vi "OP600ZP_ISO.vi"(8 "entrée d'erreur (pas d'erreur)":errorcluster, 9 "Oui":bool, 10 "reference en entrée":refnum<vi>) -> (0 "sortie d'erreur":errorcluster, 1 "ISOP":string, 2 "ISOM":string, 3 "Booléen":bool)   [LabVIEW 2020]
uses:
  VG/PackType.vi
  OP600ZP_VGConf.vi
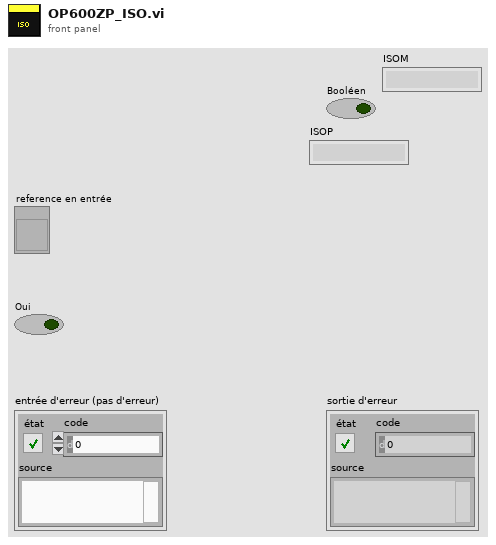
[diagram p1: front panel]
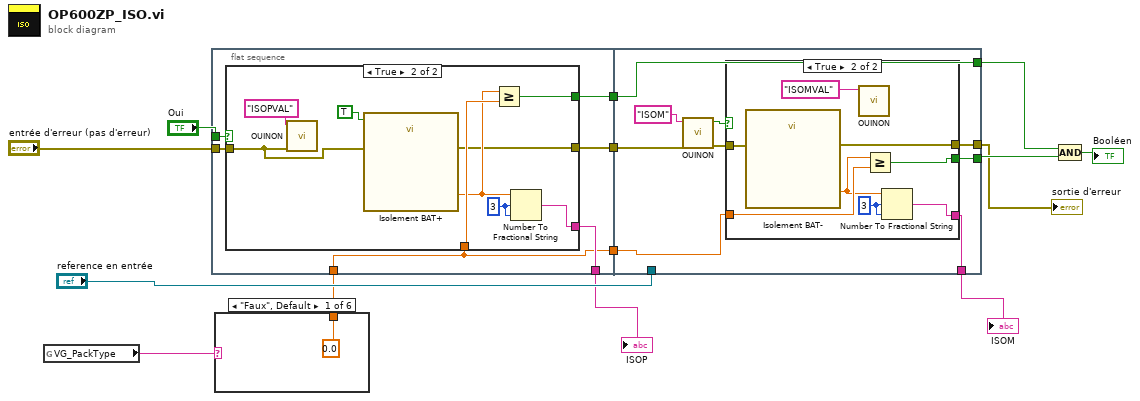
[diagram p0: block diagram]
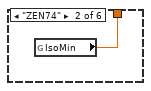
[diagram p2: hidden frame]
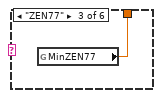
[diagram p3: hidden frame]
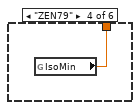
[diagram p4: hidden frame]
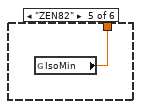
[diagram p5: hidden frame]
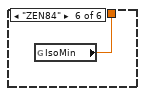
[diagram p6: hidden frame]
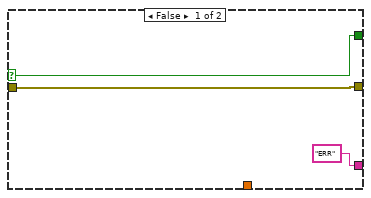
[diagram p7: hidden frame]
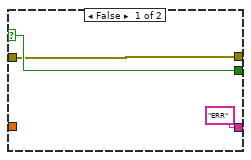
[diagram p8: hidden frame]
diagram:
  n1 = global read "PackType.vi" "VG_PackType"() -> (w5:string)
  n2 = flat-sequence {
    tunnel: [w20] -> w2
    tunnel: [w15] -> w14
    tunnel: [w19] -> w13
    tunnel: [w18] -> w12
    tunnel: "entrée d'erreur (pas d'erreur)" -> [w17]
    tunnel: "Oui" -> [w16]
    tunnel: w4 -> [w15]
    tunnel: w14 -> [w37]
    tunnel: w13 -> [w41]
    tunnel: w12 -> [w40]
    tunnel: [w35] -> w1
    tunnel: "reference en entrée" -> [_]
    tunnel: [w41] -> w7
    tunnel: [w36] -> w9
    tunnel: [w33] -> w3
    frame #0 {
      n3 = case shown="True" w16 {
        selector: w16 -> [w22 _]
        tunnel: w17 -> [w23 w24]
        tunnel: [w23 w26] -> w18
        tunnel: [w22 w29] -> w19
        tunnel: w15 -> [_ w31]
        tunnel: ["ERR" w28] -> w20
        frame False {
        }
        frame True {
          w32 = i16 3 ("largeur (-)")
          n4 = call "OUINON.vi"("errin"=w24, "image"="ISOPVAL") -> ()  [unwired: 8 in, 2 out]
          n5 = call "Isolement BAT+"("Enable"=TRUE, "error in (no error)"=w24) -> ("ISOP"=w30:dbl, "error out"=w26:errorcluster)  [unwired: 15 in, 1 out]
          n6 = Greater Or Equal?(x=w30, y=w31) -> (x >= y?=w29:bool)
          n7 = Number To Fractional String(number=w30, width (-)=w32, precision (6)=w32) -> (F-format string=w28:string)  [unwired: 1 in]
        }
      }
    }
    frame #1 {
      n8 = call "OUINON.vi"("errin"=w40, "image"="ISOM" ("IN")) -> ("error out"=w34:errorcluster, "OUI/NON"=w38:bool)  [unwired: 8 in]
      n9 = case shown="True" w38 {
        selector: w38 -> [w44 _]
        tunnel: [w42 w48] -> w33
        tunnel: [w44 w49] -> w36
        tunnel: w37 -> [_ w51]
        tunnel: ["ERR" w47] -> w35
        tunnel: w34 -> [w42 w45]
        frame False {
        }
        frame True {
          w52 = i16 3 ("largeur (-)")
          n10 = call "Isolement BAT-"("error in (no error)"=w45) -> ("ISOM"=w50:dbl, "error out"=w48:errorcluster)  [unwired: 16 in, 1 out]
          n11 = call "OUINON.vi"("image"="ISOMVAL") -> ()  [unwired: 9 in, 2 out]
          n12 = Greater Or Equal?(x=w50, y=w51) -> (x >= y?=w49:bool)
          n13 = Number To Fractional String(number=w50, width (-)=w52, precision (6)=w52) -> (F-format string=w47:string)  [unwired: 1 in]
        }
      }
    }
  }
  n14 = case shown="\"Faux\", Default" w5 {
    tunnel: [0.0 ("IsoMin") w54 w55 w56 w57 w58] -> w4
    frame "Faux", Default {
    }
    frame "ZEN74" {
      n15 = global read "OP600ZP_VGConf.vi" "IsoMin"() -> (w54:dbl)
    }
    frame "ZEN77" {
      n16 = global read "OP600ZP_VGConf.vi" "MinZEN77"() -> (w55:dbl)
    }
    frame "ZEN79" {
      n17 = global read "OP600ZP_VGConf.vi" "IsoMin"() -> (w56:dbl)
    }
    frame "ZEN82" {
      n18 = global read "OP600ZP_VGConf.vi" "IsoMin"() -> (w57:dbl)
    }
    frame "ZEN84" {
      n19 = global read "OP600ZP_VGConf.vi" "IsoMin"() -> (w58:dbl)
    }
  }
  n20 = Compound Arithmetic op=AND ("Opérateur arithmétique")(w7, w9) -> (→"Booléen":bool)
  "sortie d'erreur" <- w3
  "ISOP" <- w2
  "ISOM" <- w1
